vi "DSF.Execution.Runtime.Plugin Manager.Initialize.vi"(8 "error in (no error)":errorcluster, 10 "Plugins folder":path, 11 "Plugin Manager in":refnum<class "Plugin Manager.lvclass">) -> (0 "error out":errorcluster, 3 "Plugin Manager out":refnum<class "Plugin Manager.lvclass">)   [LabVIEW 2016, in "DSF.Engine.lvlib" / "Plugin Manager.lvclass"]
uses:
  Plugin Manager.lvclass
  Plugin Manager.lvclass/Plugin Manager.ctl
  <vilib>/Utility/libraryn.llb/Check if File or Folder Exists.vi
  <vilib>/Utility/libraryn.llb/Recursive File List.vi
  <vilib>/Utility/LVClass/Get LV Class Default Value.vi
  Plugin/DSF.Engine.Runtime.Plugin.lvclass
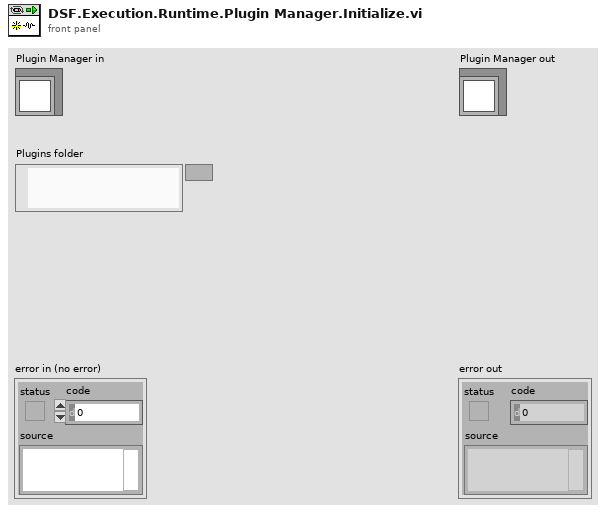
[diagram p1: front panel]
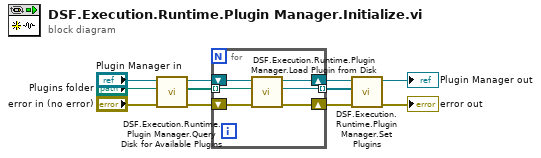
[diagram p0: block diagram]
diagram:
  n1 = call "DSF.Execution.Runtime.Plugin Manager.Query Disk for Available Plugins.vi"("error in (no error)"="error in (no error)", "Plugins folder"="Plugins folder", "Plugin Manager in"="Plugin Manager in") -> ("error out"=w6:errorcluster, "Plugin paths"=w5:path[], "Plugin Manager out"=w8:refnum<class "Plugin Manager.lvclass">)  [unwired: 6 in]
  n2 = for {
    shift-right: [w16] -> w7
    shift-left: w8 -> [w17]
    shift-right: [w15] -> w3
    shift-left: w6 -> [w14]
    tunnel: w5 -> [w13] mode=indexing
    tunnel: [w12] -> w4 mode=indexing
    n3 = call "DSF.Execution.Runtime.Plugin Manager.Load Plugin from Disk.vi"("error in (no error)"=w14, "path to Plugin"=w13, "Plugin Manager in"=w17) -> ("error out"=w15:errorcluster, "Plugin"=w12:refnum<class "DSF.Engine.Runtime.Plugin.lvclass">, "Plugin Manager out"=w16:refnum<class "Plugin Manager.lvclass">)  [unwired: 6 in]
  }
  n4 = call "DSF.Execution.Runtime.Plugin Manager.Set Plugins.vi"("error in (no error)"=w3, "Plugins"=w4, "Plugin Manager in"=w7) -> ("error out"=→"error out":errorcluster, "Plugin Manager out"=→"Plugin Manager out":refnum<class "Plugin Manager.lvclass">)  [unwired: 7 in]
